vi "HFRR ADV v03.vi"() -> ()   [LabVIEW 2025] (continued)
            n287 = property on="Service Password Log" class="Str"("Visible"=FALSE) -> ()  [unwired: 2 in, 2 out]
            "Service Password enable" <- w384
          }
        }
      }
      event "Sign In": Value Change {
        w386 = FALSE ("Visible")
        n288 = event-data() -> ()  [unwired: 1 in, 6 out]
        n289 = property on="About" class="Clust (strict)"("Visible"=w386) -> ()  [unwired: 2 in, 2 out]
        n290 = property on="Password 3" class="Clust (strict)"("Visible"=w386) -> ()  [unwired: 2 in, 2 out]
        n291 = property on="Service Password Log" class="Str"("Visible"=FALSE) -> ()  [unwired: 2 in, 2 out]
      }
      event "Info": Value Change {
        n292 = event-data() -> ()  [unwired: 1 in, 6 out]
        n293 = local read "Info"() -> (w388:bool)
        n294 = case shown="False" w388 {
          frame False {
            n295 = property on="About" class="Clust (strict)"("Visible"=FALSE) -> ()  [unwired: 2 in, 2 out]
          }
          frame True {
            n296 = property on="About" class="Clust (strict)"("Visible"=TRUE) -> ()  [unwired: 2 in, 2 out]
          }
        }
      }
      event "Calibration": Value Change {
        n297 = event-data() -> ()  [unwired: 1 in, 6 out]
        n298 = local read "Calibration"() -> (w392:bool)
        n299 = case shown="False" w392 {
          frame False {
            n300 = property on="Calibration 2" class="TabCtl (strict)"("Visible"=FALSE) -> ()  [unwired: 2 in, 2 out]
            n301 = local write "Cal Password"("" ("Cal Password")) -> ()
          }
          frame True {
            n302 = property on="Calibration 2" class="TabCtl (strict)"("Visible"=TRUE) -> ()  [unwired: 2 in, 2 out]
            n303 = local write "Cal Password"("" ("Cal Password")) -> ()
          }
        }
        n304 = property on="Wrong Password" class="Str"("Visible"=FALSE) -> ()  [unwired: 2 in, 2 out]
      }
      event "Cal Password": Value Change {
        n305 = event-data() -> ()  [unwired: 1 in, 6 out]
        n306 = local read "Cal Password"() -> (w400:string)
        n307 = call <vilib>:"Trim Whitespace.vi"("string"=w400) -> ("trimmed string"=w399:string)  [unwired: 1 in]
        n308 = Equal?(x=w399, y="Cal@321") -> (x = y?=w397:bool)
        n309 = case shown="True" w397 {
          frame False {
            n310 = property on="Wrong Password" class="Str"("Visible"=TRUE) -> ()  [unwired: 2 in, 2 out]
          }
          frame True {
            n311 = property on="Wrong Password" class="Str"("Visible"=FALSE) -> ()  [unwired: 2 in, 2 out]
            n312 = local write "Main Tab"(T2."About" ("Main Tab")) -> ()
            n313 = local write "Cal Password"("" ("Cal Password")) -> ()
            n314 = local write "Main Dashboard Buttons"(T1."About" ("Main Dashboard Buttons")) -> ()
            n315 = local write "Tab Control 5"(T7."Temperature Calibration" ("Tab Control 5")) -> ()
            n316 = property on="Calibration 2" class="TabCtl (strict)"("Visible"=FALSE) -> ()  [unwired: 2 in, 2 out]
            n317 = property on="Tab Control 5" class="TabCtl (strict)"("Tabs Visible?"=FALSE ("Page Labels Display Visible?")) -> ()  [unwired: 2 in, 2 out]
            n318 = local write "Calibration"(FALSE ("Calibration")) -> ()
          }
        }
      }
      event "Quit": Value Change {
        n319 = event-data() -> ()  [unwired: 1 in, 6 out]
      }
    }
    n320 = Wait (ms)(milliseconds to wait=u32 100) -> ()  [unwired: 1 out]
  }
  n321 = local write "Auto stop temp"(w12) -> ()
  n322 = local write "main tab sub"(enum32{"Page 1", "Page 2"}."Page 1" ("main tab sub")) -> ()
  n323 = local write "USERNAME"(w31) -> ()
  n324 = local write "Main Tab"(T2."HOME" ("Main Tab")) -> ()
  n325 = local write "USER ID"(w31) -> ()
  n326 = property on="Auto Scar Check  2" class="Clust (strict)"("Visible"=w12) -> (error out=w16:errorcluster)  [unwired: 2 in, 1 out]
  n327 = property on="Quit" class="Bool (strict)"("Value"=FALSE ("Quit")) -> (error out=w33:errorcluster)  [unwired: 2 in, 1 out]
  n328 = while {
    shift-right: [w412] -> _
    shift-left: "Enum - Selector" -> [w413]
    stop <- w414 stop-if-true
    # "Auto Start Logic Loop"
    n329 = case shown="\"close\"" w413 {
      tunnel: [w417 w423 w434 w466 w497 Auto_Start_enum."Exit" ("Enum - Selector") Auto_Start_enum."Init" ("Enum - Selector")] -> w412
      frame "Init", Default {
        n330 = local read "Auto Start Test"() -> (w416:bool)
        n331 = Select(t=Auto_Start_enum."Humidity & Temperature On" ("Enum - Selector"), s=w416, f=Auto_Start_enum."Init") -> (s? t:f=w417:T10)
      }
      frame "Humidity & Temperature On" {
        n332 = flat-sequence {
          tunnel: [Auto_Start_enum."Reach point" ("Enum - Selector")] -> w420
          frame #0 {
            w424 = T13."Disabled and Grayed Out" ("Disabled")
            w425 = TRUE ("Heater Button")
            n333 = property on="Humidity" class="Bool (strict)"("DisabledEnum"=w424) -> ()  [unwired: 2 in, 2 out]
            n334 = property on="Heater Button" class="Bool (strict)"("DisabledEnum"=w424) -> ()  [unwired: 2 in, 2 out]
            n335 = local write "Heater Button"(w425) -> ()
            n336 = local write "Humidity"(w425) -> ()
          }
          frame #1 {
            n337 = Wait (ms)(milliseconds to wait=u32 1000) -> ()  [unwired: 1 out]
          }
          frame #2 {
            w427 = TRUE ("Reach point temp")
            n338 = local write "Reach point Humidity"(w427) -> ()
            n339 = local write "Reach point temp"(w427) -> ()
          }
        }
        n340 = local read "Auto Start Test"() -> (w422:bool)
        n341 = Not(x=w422) -> (.not. x?=w421:bool)
        n342 = Select(t=Auto_Start_enum."close", s=w421, f=w420) -> (s? t:f=w423:T10)
      }
      frame "Reach point" {
        w435 = TRUE ("PAUSE")
        w443 = 1.0 ("y")
        w446 = 1.0 ("y")
        n343 = local read "Set Temperature:"() -> (w447:dbl)
        n344 = local read "Set Humidity:"() -> (w442:dbl)
        n345 = local read "Humidity ( %RH )"() -> (w448:dbl)
        n346 = Add(x=w447, y=w446) -> (x+y=w445:dbl)
        n347 = Subtract(x=w447, y=w446) -> (x-y=w444:dbl)
        n348 = Add(x=w442, y=w443) -> (x+y=w441:dbl)
        n349 = Subtract(x=w442, y=w443) -> (x-y=w440:dbl)
        n350 = local read "TEMP"() -> (w449:dbl)
        n351 = In Range and Coerce(upper limit=w441, x=w448, lower limit=w440) -> (In Range?=w429:bool)  [unwired: 1 out]
        n352 = In Range and Coerce(upper limit=w445, x=w449, lower limit=w444) -> (In Range?=w430:bool)  [unwired: 1 out]
        n353 = case shown="True" w429 {
          frame False {
          }
          frame True {
            n354 = case shown="True" "Reach point Humidity" {
              selector: "Reach point Humidity" -> [_ w455]
              frame False {
              }
              frame True {
                n355 = local read "EVENT LOG"() -> (w452:string)
                n356 = Not(x=w455) -> (.not. x?=w454:bool)
                n357 = local write "Reach point Humidity"(w454) -> ()
                n358 = call "Event Log.vi"("Content"="Target Humidity reached", "EVENT LOG"=w452) -> ("EVENT LOG"=w453:string)  [unwired: 8 in, 1 out]
                n359 = local write "EVENT LOG"(w453) -> ()
              }
            }
          }
        }
        n360 = case shown="True" w430 {
          frame False {
          }
          frame True {
            n361 = case shown="True" "Reach point temp" {
              selector: "Reach point temp" -> [_ w461]
              frame False {
              }
              frame True {
                n362 = local read "EVENT LOG"() -> (w458:string)
                n363 = Not(x=w461) -> (.not. x?=w460:bool)
                n364 = local write "Reach point temp"(w460) -> ()
                n365 = call "Event Log.vi"("Content"="Target Temperature reached", "EVENT LOG"=w458) -> ("EVENT LOG"=w459:string)  [unwired: 8 in, 1 out]
                n366 = local write "EVENT LOG"(w459) -> ()
              }
            }
          }
        }
        n367 = local read "Auto Start Test"() -> (w433:bool)
        n368 = And(x=w430, y=w429) -> (x .and. y?=w439:bool)
        n369 = Select(t=Auto_Start_enum."Maintain Stage" ("Enum - Selector"), s=w439, f=Auto_Start_enum."Reach point" ("Enum - Selector")) -> (s? t:f=w436:T10)
        n370 = Not(x=w433) -> (.not. x?=w432:bool)
        n371 = Select(t=Auto_Start_enum."close", s=w432, f=w436) -> (s? t:f=w434:T10)
        n372 = call "ELAPSED TIMER VI.vi"("RESET"=w435, "PAUSE"=w435) -> ()  [unwired: 7 in, 3 out]
      }
      frame "Maintain Stage" {
        w475 = 2.0 ("y")
        w474 = 1.0 ("y")
        # "Humidity and  temperatures Set Point  have been reached"
        n373 = local read "Set Temperature:"() -> (w481:dbl)
        n374 = local read "Set Humidity:"() -> (w478:dbl)
        n375 = local read "Humidity ( %RH )"() -> (w482:dbl)
        n376 = Add(x=w481, y=w474) -> (x+y=w480:dbl)
        n377 = Subtract(x=w481, y=w474) -> (x-y=w479:dbl)
        n378 = local read "TEMP"() -> (w483:dbl)
        n379 = Add(x=w478, y=w475) -> (x+y=w477:dbl)
        n380 = Subtract(x=w478, y=w475) -> (x-y=w476:dbl)
        n381 = In Range and Coerce(upper limit=w480, x=w483, lower limit=w479) -> (In Range?=w473:bool)  [unwired: 1 out]
        n382 = In Range and Coerce(upper limit=w477, x=w482, lower limit=w476) -> (In Range?=w472:bool)  [unwired: 1 out]
        n383 = And(x=w473, y=w472) -> (x .and. y?=w471:bool)
        n384 = Not(x=w471) -> (.not. x?=w470:bool)
        n385 = call "ELAPSED TIMER VI.vi"("TARGET"=60.0, "RESET"=w470, "PAUSE"=FALSE) -> ("ELAPSED INDICATION"=w467:bool)  [unwired: 6 in, 2 out]
        n386 = case shown="True" w467 {
          tunnel: w467 -> [_ w486]
          tunnel: [Auto_Start_enum."Maintain Stage" ("Enum - Selector") w485] -> w465
          frame False {
          }
          frame True {
            n387 = stacked-sequence {
              tunnel: w486 -> [_ _ _ _ _]
              tunnel: [_ _ _ _ Auto_Start_enum."Start Stage" ("Enum - Selector")] -> w485
              frame #0 {
                n388 = local read "EVENT LOG"() -> (w488:string)
                n389 = call "Event Log.vi"("Content"="Humidity and temperature set point has stabilized.", "EVENT LOG"=w488) -> ("EVENT LOG"=w489:string)  [unwired: 8 in, 1 out]
                n390 = local write "EVENT LOG"(w489) -> ()
              }
              frame #1 {
                n391 = Wait (ms)(milliseconds to wait=u32 100) -> ()  [unwired: 1 out]
              }
              frame #2 {
                n392 = local read "EVENT LOG"() -> (w492:string)
                n393 = call "Event Log.vi"("Content"="Auto Test Started", "EVENT LOG"=w492) -> ("EVENT LOG"=w493:string)  [unwired: 8 in, 1 out]
                n394 = local write "EVENT LOG"(w493) -> ()
              }
              frame #3 {
                w494 = TRUE ("RUN")
                n395 = local write "RUN"(w494) -> ()
                "Auto Start Temp" <- w494
              }
              frame #4 {
              }
            }
          }
        }
        n396 = local read "Auto Start Test"() -> (w464:bool)
        n397 = Not(x=w464) -> (.not. x?=w463:bool)
        n398 = Select(t=Auto_Start_enum."close", s=w463, f=w465) -> (s? t:f=w466:T10)
      }
      frame "Start Stage" {
        w496 = TRUE ("PAUSE")
        n399 = local read "Auto Start Test"() -> (w501:bool)
        n400 = Not(x=w501) -> (.not. x?=w500:bool)
        n401 = Select(t=Auto_Start_enum."close" ("Enum - Selector"), s=w500, f=Auto_Start_enum."Start Stage" ("Enum - Selector")) -> (s? t:f=w497:T10)
        n402 = call "ELAPSED TIMER VI.vi"("RESET"=w496, "PAUSE"=w496) -> ()  [unwired: 7 in, 3 out]
      }
      frame "close" {
        w502 = FALSE ("Heater Button")
        n403 = local write "RUN"(w502) -> ()
        n404 = local write "Heater Button"(w502) -> ()
        n405 = local write "Humidity"(w502) -> ()
        n406 = local write "Auto Start Test"(w502) -> ()
      }
      frame "Exit" {
      }
    }
    n407 = Wait (ms)(milliseconds to wait=u32 100) -> ()  [unwired: 1 out]
    n408 = local read "Quit"() -> (w414:bool)
  }
  n409 = while {
    stop <- w531 stop-if-true
    w514 = errorcluster {"status"=FALSE, "code"=0, "source"=""} ("error in (no error) 3")
    # "this loop is for manual report generation"
    n410 = local read "Confirm Measrurement"() -> (w513:bool)
    n411 = case shown="True" w513 {
      selector: w513 -> [_ w621]
      tunnel: errorcluster {"status"=FALSE, "code"=0, "source"=""} ("error in (no error) 3") -> [_ w622]
      tunnel: [_ w620] -> _
      frame False {
      }
      frame True {
        n412 = stacked-sequence {
          tunnel: w622 -> [_ w655 _]
          tunnel: w621 -> [_ _ w762]
          tunnel: [_ w643 _] -> w620
          frame #0 {
            n413 = String To Path(string="C:\\LAB-IQ\\Image Calibrate v01.dcf") -> (path=w625:path)
            n414 = Open/Create/Replace File ("Open File")(file path (use dialog)=w625) -> (refnum out=w626:refnum<file>)  [unwired: 5 in, 2 out]
            n415 = for {
              N: 4 -> [_]
              tunnel: w626 -> [w632]
              i -> [w628]
              n416 = Read from Text File ("Read File")(file (use dialog)=w632) -> (text=w633:string)  [unwired: 3 in, 3 out]
              n417 = String Subset(string=w633, offset (0)=6, length (rest)=10 ("length (rest)")) -> (substring=w629:string)
              n418 = Fract/Exp String To Number(string=w629) -> (number=w627:dbl)  [unwired: 3 in, 1 out]
              n419 = case shown="3" w628 {
                tunnel: w627 -> [w634 w635 _ w636 _]
                frame 0 {
                  n420 = local write "5x Gain"(w634) -> ()
                }
                frame 1 {
                  n421 = local write "10x Gain"(w635) -> ()
                }
                frame 2 {
                }
                frame 3 {
                  n422 = local write "100x gain"(w636) -> ()
                }
                frame 4, Default {
                }
              }
            }
          }
          frame #1 {
            n423 = local read "TEST STANDARD"() -> (w638:T3)
            n424 = case shown="\"ISO 12156\"" w638 {
              tunnel: ["ASTM D6079" "ISO 12156"] -> w637
              frame "ASTM D6079", Default {
              }
              frame "ISO 12156" {
              }
            }
            n425 = call "IMAGE ANALYSIS.vi"("Enum"=POST_ANALYSIS_ENUM."GET MEASUREMENTS", "error in"=w655) -> ("error out"=w662:errorcluster)  [unwired: 8 in, 1 out]
            n426 = local read "Magnification :"() -> (w648:string)
            n427 = call "Stall Data Flow.vim"("value in"=w662, "milliseconds to wait"=u32 1000) -> ("value out"=w661:errorcluster)  [unwired: 1 out]
            n428 = local read "Test File List :"() -> (w659:string)
            n429 = case shown="\"10x\"" w648 {
              tunnel: [w698 w699] -> w646
              frame "5x", Default {
                n430 = local read "5x Gain"() -> (w698:dbl)
              }
              frame "10x" {
                # "5x"
                n431 = local read "10x Gain"() -> (w699:dbl)
              }
            }
            n432 = call "IMAGE ANALYSIS.vi"("Enum"=POST_ANALYSIS_ENUM."READ", "error in"=w661) -> ("error out"=w658:errorcluster, "data out"=w649:string)  [unwired: 8 in]
            n433 = Match Pattern(string=w649, regular expression="\"type\": ") -> (after substring=w653:string)  [unwired: 1 in, 3 out]
            n434 = call "IMAGE PATH CREATION PY.vi"("error in (no error)"=w658, "File Name :"=w659) -> ("error out"=w657:errorcluster, "File Path"=w645:path, "File Path String:"=w640:string)  [unwired: 7 in]
            n435 = Match Pattern(string=w653, regular expression=",") -> (before substring=w639:string)  [unwired: 1 in, 3 out]
            n436 = local read "Calibration Tab"() -> (w642:enum32{"Measrument", "Calibrate"})
            n437 = call "Stall Data Flow.vim"("value in"=w657, "milliseconds to wait"=u32 250) -> ("value out"=w641:errorcluster)  [unwired: 1 out]
            n438 = Equal?(x=w639, y="\"rectangle\"") -> (x = y?=w650:bool)
            n439 = case shown="False" w650 {
              tunnel: w649 -> [w704 w759]
              tunnel: w646 -> [_ w750]
              tunnel: cluster{"major":dbl, "minor":dbl, "average":dbl} {"major"=0.0, "minor"=0.0, "average"=0.0} -> [w702 w746]
              tunnel: [w701 w743] -> w644
              tunnel: w639 -> [w703 _]
              tunnel: w646 -> [w700 _]
              frame False {
                n440 = Equal?(x=w703, y="\"line\"") -> (x = y?=w705:bool)
                n441 = case shown="True" w705 {
                  tunnel: w704 -> [_ w720]
                  tunnel: w702 -> [w707 w719]
                  tunnel: [w707 w717] -> w701
                  tunnel: w700 -> [_ w716]
                  frame False {
                  }
                  frame True {
                    w715 = 0.0 ("Major Axis")
                    n442 = Match Pattern(string=w720, regular expression="\"length_px\":") -> (after substring=w718:string)  [unwired: 1 in, 3 out]
                    n443 = property on="Major Axis" class="DigNum (strict)"("Caption.Text"="") -> ()  [unwired: 2 in, 2 out]
                    n444 = property on="Minor Axis" class="DigNum (strict)"("Caption.Text"="") -> ()  [unwired: 2 in, 2 out]
                    n445 = property on="Average" class="DigNum (strict)"("Caption.Text"="Line") -> ()  [unwired: 2 in, 2 out]
                    n446 = Fract/Exp String To Number(string=w718, default (0 dbl)=0.0 ("default (0 DBL)")) -> (number=w714:dbl)  [unwired: 2 in, 1 out]
                    "Pixel Value" <- w714
                    n447 = Multiply(x=w714, y=w716) -> (x*y=w727:dbl)
                    n448 = Multiply(x=w727, y=1000.0) -> (x*y=w710:dbl)
                    n449 = Divide(x=w710, y=1000.0) -> (x/y=w713:dbl)
                    n450 = local write "Measurment (mm)"(w713) -> ()
                    n451 = Bundle By Name(cluster=w719, "average"=w710) -> (w717:cluster{"major":dbl, "minor":dbl, "average":dbl})
                    n452 = Number To Fractional String(number=w710, precision (6)=i16 1) -> (F-format string=w709:string)  [unwired: 2 in]
                    n453 = local write "Minor Axis"(w715) -> ()
                    n454 = local write "Major Axis"(w715) -> ()
                    n455 = Fract/Exp String To Number(string=w709) -> (number=w708:dbl)  [unwired: 3 in, 1 out]
                    n456 = local write "Average"(w708) -> ()
                  }
                }
              }
              frame True {
                w747 = 1000.0 ("y")
                w753 = 0.0 ("default (0 DBL)")
                n457 = Match Pattern(string=w759, regular expression=" \"width_px\":") -> (after substring=w757:string)  [unwired: 1 in, 3 out]
                n458 = Match Pattern(string=w757, regular expression="\"height_px\":") -> (before substring=w755:string, after substring=w754:string)  [unwired: 1 in, 2 out]
                n459 = Fract/Exp String To Number(string=w755, default (0 dbl)=w753) -> (number=w752:dbl)  [unwired: 2 in, 1 out]
                n460 = Fract/Exp String To Number(string=w754, default (0 dbl)=w753) -> (number=w751:dbl)  [unwired: 2 in, 1 out]
                n461 = Multiply(x=w752, y=w750) -> (x*y=w749:dbl)
                n462 = Multiply(x=w751, y=w750) -> (x*y=w748:dbl)
                n463 = Multiply(x=w749, y=w747) -> (x*y=w733:dbl)
                n464 = Multiply(x=w748, y=w747) -> (x*y=w731:dbl)
                n465 = Add(x=w733, y=w731) -> (x+y=w745:dbl)
                n466 = property on="Major Axis" class="DigNum (strict)"("Caption.Text"="Major Axis") -> ()  [unwired: 2 in, 2 out]
                n467 = property on="Minor Axis" class="DigNum (strict)"("Caption.Text"="Minor Axis") -> ()  [unwired: 2 in, 2 out]
                n468 = property on="Average" class="DigNum (strict)"("Caption.Text"="Average") -> ()  [unwired: 2 in, 2 out]
                n469 = Divide(x=w745, y=2.0) -> (x/y=w729:dbl)
                n470 = Bundle By Name(cluster=w746, "major"=w733, "minor"=w731, "average"=w729) -> (w743:cluster{"major":dbl, "minor":dbl, "average":dbl})
                n471 = Number To Fractional String(number=w731, precision (6)=i16 1) -> (F-format string=w738:string)  [unwired: 2 in]
                n472 = Number To Fractional String(number=w729, precision (6)=i16 1) -> (F-format string=w739:string)  [unwired: 2 in]
                n473 = Number To Fractional String(number=w733, precision (6)=i16 1) -> (F-format string=w737:string)  [unwired: 2 in]
                n474 = Fract/Exp String To Number(string=w738) -> (number=w730:dbl)  [unwired: 3 in, 1 out]
                n475 = Fract/Exp String To Number(string=w739) -> (number=w728:dbl)  [unwired: 3 in, 1 out]
                n476 = Fract/Exp String To Number(string=w737) -> (number=w732:dbl)  [unwired: 3 in, 1 out]
                n477 = local write "Major Axis"(w732) -> ()
                n478 = local write "Average"(w728) -> ()
                n479 = local write "Minor Axis"(w730) -> ()
              }
            }
            n480 = case shown="\"Measrument\", Default" w642 {
              tunnel: w645 -> [w672 _]
              tunnel: w644 -> [w671 _]
              tunnel: [w668 w697] -> w643
              tunnel: w641 -> [w670 w697]
              tunnel: w640 -> [w669 _]
              tunnel: w637 -> [w667 _]
              frame "Measrument", Default {
                n481 = stacked-sequence {
                  tunnel: w672 -> [w690 _]
                  tunnel: w671 -> [w688 _]
                  tunnel: w670 -> [w686 _]
                  tunnel: w669 -> [w685 _]
                  tunnel: [w680 _] -> w668
                  tunnel: w667 -> [w673 _]
                  frame #0 {
                    n482 = call "IMAGE ANALYSIS.vi"("Enum"=POST_ANALYSIS_ENUM."SAVE IMAGE", "error in"=w686, "IMAGE FILE PATH"=w685) -> ("error out"=w684:errorcluster)  [unwired: 7 in, 1 out]
                    n483 = call "Stall Data Flow.vim"("value in"=w684, "milliseconds to wait"=u32 1000) -> ("value out"=w675:errorcluster)  [unwired: 1 out]
                    n484 = local read "Test File List :"() -> (w692:string)
                    n485 = call "IMAGE ANALYSIS.vi"("Enum"=POST_ANALYSIS_ENUM."MINIMIZE UI", "error in"=w675) -> ("error out"=w682:errorcluster)  [unwired: 8 in, 1 out]
                    n486 = Bundle By Name(cluster=T18 {"File Name"="", "Test Method"="", "Operator"="", "Fuel Description"="", "Date and time"=""} ("Main Ref"), "Test Method"=w673, "File Name"=w692) -> (w693:T18)
                    n487 = call "Stall Data Flow.vim"("value in"=w682, "milliseconds to wait"=u32 1500) -> ("value out"=w677:errorcluster)  [unwired: 1 out]
                    n488 = call "duf file read.vi"("error in (no error)"=w677, "Main Ref"=w693) -> ("error out"=w691:errorcluster, "Main Ref 2"=w689:T18)  [unwired: 8 in]
                    n489 = call "DETECTION REPORT for manual.vi"("error in (no error)"=w691, "return value 3"=w688, "Image File Path"=w690, "Main Ref"=w689) -> ("error out"=w687:errorcluster)  [unwired: 7 in]
                    n490 = call <vilib>:"Clear Errors.vi"("error in (no error)"=w687) -> ("error out"=w678:errorcluster)  [unwired: 5 in, 1 out]
                    n491 = call "IMAGE ANALYSIS.vi"("Enum"=POST_ANALYSIS_ENUM."MINIMIZE UI", "error in"=w678) -> ("error out"=w680:errorcluster)  [unwired: 8 in, 1 out]
                  }
                  frame #1 {
                    n492 = local write "Main Tab"(T2."HOME" ("Main Tab")) -> ()
                    n493 = local write "Main Dashboard Buttons"(T1."Home" ("Main Dashboard Buttons")) -> ()
                  }
                }
              }
              frame "Calibrate" {
              }
            }
          }
          frame #2 {
            n494 = Not(x=w762) -> (.not. x?=w761:bool)
            n495 = local write "Confirm Measrurement"(w761) -> ()
            n496 = local read "Calibration Tab"() -> (w760:enum32{"Measrument", "Calibrate"})
            n497 = case shown="\"Measrument\", Default" w760 {
              frame "Measrument", Default {
                n498 = local write "Main Tab"(T2."HOME" ("Main Tab")) -> ()
              }
              frame "Calibrate" {
              }
            }
          }
        }
      }
    }
    n499 = local read "Humidity"() -> (w505:bool)
    n500 = local read "Save Change"() -> (w510:bool)
    n501 = local read "Calibrate"() -> (w511:bool)
    n502 = local read "Auto Start Test"() -> (w506:bool)
    n503 = case shown="True" w511 {
      selector: w511 -> [_ w618]
      frame False {
      }
      frame True {
        n504 = Not(x=w618) -> (.not. x?=w617:bool)
        n505 = local write "Calibrate"(w617) -> ()
        n506 = local write "Calibration Tab"(enum32{"Measrument", "Calibrate"}."Calibrate" ("Calibration Tab")) -> ()
      }
    }
    n507 = case shown="True" w510 {
      selector: w510 -> [_ w562]
      frame False {
      }
      frame True {
        n508 = stacked-sequence {
          tunnel: w562 -> [_ _ _ _ w616]
          frame #0 {
            n509 = call "IMAGE ANALYSIS.vi"("Enum"=POST_ANALYSIS_ENUM."HIDE UI") -> ()  [unwired: 9 in, 2 out]
          }
          frame #1 {
            n510 = local read "100x gain"() -> (w564:dbl)
            n511 = local read "10x Gain"() -> (w565:dbl)
            n512 = local read "5x Gain"() -> (w566:dbl)
            n513 = Number To Fractional String(number=w565, width (-)=i16 4, precision (6)=i16 7) -> (F-format string=w587:string)  [unwired: 1 in]
            n514 = Number To Fractional String(number=0.0, width (-)=i16 4, precision (6)=i16 7) -> (F-format string=w582:string)  [unwired: 1 in]
            n515 = Number To Fractional String(number=w564, width (-)=i16 4, precision (6)=i16 7) -> (F-format string=w570:string)  [unwired: 1 in]
            n516 = Number To Fractional String(number=w566, width (-)=i16 10 ("precision (6)"), precision (6)=i16 7) -> (F-format string=w596:string)  [unwired: 1 in]
            n517 = Concatenate Strings("[CH1]" ("string"), w596, " - 5x Gain" ("string"), "\r") -> (w586:string)
            n518 = Concatenate Strings("[CH2]" ("string"), w587, " - 10x Gain" ("string"), "\r") -> (w585:string)
            n519 = Concatenate Strings("[CH3]" ("string"), w582, " - 20x Gain" ("string"), "\r") -> (w576:string)
            n520 = Concatenate Strings("[CH4]" ("string"), w570, " - 100x Gain" ("string"), "\r") -> (w569:string)
            n521 = String To Path(string="C:\\LAB-IQ\\Image Calibrate v01.dcf") -> (path=w599:path)
            n522 = Concatenate Strings(w586, w585, w576, w569) -> (w584:string)
            n523 = call <vilib>:"Write Characters To File.vi"("append to file? (new file:F)"=FALSE, "character string"=w584, "file path (dialog if empty)"=w599) -> ()  [unwired: 2 in, 1 out]
          }
          frame #2 {
            n524 = String To Path(string="C:\\LAB-IQ\\Image Calibrate v01.dcf") -> (path=w602:path)
            n525 = Open/Create/Replace File ("Open File")(file path (use dialog)=w602) -> (refnum out=w603:refnum<file>)  [unwired: 5 in, 2 out]
            n526 = for {
              N: 4 -> [_]
              tunnel: w603 -> [w609]
              i -> [w605]
              n527 = Read from Text File ("Read File")(file (use dialog)=w609) -> (text=w610:string)  [unwired: 3 in, 3 out]
              n528 = String Subset(string=w610, offset (0)=6, length (rest)=10 ("length (rest)")) -> (substring=w606:string)
              n529 = Fract/Exp String To Number(string=w606) -> (number=w604:dbl)  [unwired: 3 in, 1 out]
              n530 = case shown="3" w605 {
                tunnel: w604 -> [w611 w612 _ w613 _]
                frame 0 {
                  n531 = local write "5x Gain"(w611) -> ()
                }
                frame 1 {
                  n532 = local write "10x Gain"(w612) -> ()
                }
                frame 2 {
                }
                frame 3 {
                  n533 = local write "100x gain"(w613) -> ()
                }
                frame 4, Default {
                }
              }
            }
          }
          frame #3 {
            n534 = call "IMAGE ANALYSIS.vi"("Enum"=POST_ANALYSIS_ENUM."SHOW UI") -> ()  [unwired: 9 in, 2 out]
          }
          frame #4 {
            n535 = Not(x=w616) -> (.not. x?=w615:bool)
            n536 = local write "Save Change"(w615) -> ()
          }
        }
      }
    }
    n537 = case shown="False" w506 {
      tunnel: w505 -> [w532 _]
      frame False {
        n538 = case shown="True" w532 {
          frame False {
          }
          frame True {
            n539 = local read "Set Humidity:"() -> (w536:dbl)
            n540 = local read "Set Humidity:"() -> (w539:dbl)
            n541 = local read "Humidity ( %RH )"() -> (w540:dbl)
            n542 = Subtract(x=w536, y=2.0) -> (x-y=w534:dbl)
            n543 = Add(x=w539, y=2.0) -> (x+y=w535:dbl)
            n544 = In Range and Coerce(upper limit=w535, x=w540, lower limit=w534) -> (In Range?=w533:bool)  [unwired: 1 out]
            n545 = case shown="True" w533 {
              frame False {
              }
              frame True {
                n546 = case shown="False" "Manual Humididty Reached" {
                  selector: "Manual Humididty Reached" -> [_ w543]
                  frame False {
                  }
                  frame True {
                    n547 = Not(x=w543) -> (.not. x?=w542:bool)
                    n548 = local write "Manual Humididty Reached"(w542) -> ()
                    n549 = local read "EVENT LOG"() -> (w545:string)
                    n550 = call "Event Log.vi"("Content"="Target Humidity reached", "EVENT LOG"=w545) -> ("EVENT LOG"=w544:string)  [unwired: 8 in, 1 out]
                    n551 = local write "EVENT LOG"(w544) -> ()
                  }
                }
              }
            }
          }
        }
      }
      frame True {
        n552 = local write "Manual Humididty Reached"(TRUE ("Manual Humididty Reached")) -> ()
      }
    }
    n553 = local read "Cap Live Image"() -> (w526:bool)
    n554 = local read "SCAR MEASURMENT"() -> (w529:enum32{"Auto Scar", "Manual Scar"})
    n555 = Wait (ms)(milliseconds to wait=u32 250) -> ()  [unwired: 1 out]
    n556 = Equal?(x=w529, y=enum32{"Auto Scar", "Manual Scar"}."Manual Scar" ("SCAR MEASURMENT")) -> (x = y?=w527:bool)
    n557 = And(x=w527, y=w526) -> (x .and. y?=w525:bool)
    n558 = case shown="True" w525 {
      selector: w525 -> [_ w841]
      frame False {
      }
      frame True {
        n559 = stacked-sequence {
          tunnel: [_ _ _ w856 _] -> _
          tunnel: w841 -> [_ _ _ _ w862]
          frame #0 {
            w842 = 0.0
            n560 = local write "Major Axis"(w842) -> ()
            n561 = local write "Minor Axis"(w842) -> ()
            n562 = local write "Average"(w842) -> ()
          }
          frame #1 {
            n563 = call "CAMERA LIVE FEED FGV.vi"("Enum - Menu"=CAMERA_LIVE_FEED_ENUM."CAMERA MINIMIZE") -> ()  [unwired: 9 in, 2 out]
          }
          frame #2 {
            n564 = local read "FILE 3"() -> (w850:string)
            n565 = call <vilib>:"Trim Whitespace.vi"("string"="C:\\LAB-IQ\\images\\") -> ("trimmed string"=w852:string)  [unwired: 1 in]
            n566 = String To Path(string=w852) -> (path=w851:path)
            n567 = Concatenate Strings(w850, ".png" ("string")) -> (w849:string)
            n568 = Build Path(base path=w851, name or relative path=w849) -> (appended path=w847:path)
            n569 = Path To String(path=w847) -> (string=w846:string)
            n570 = call "CAMERA LIVE FEED FGV.vi"("Enum - Menu"=CAMERA_LIVE_FEED_ENUM."CAMERA SAVE", "Image Path"=w846) -> ("error out"=w844:errorcluster)  [unwired: 8 in, 1 out]
            n571 = case shown="No Error" w844 {
              frame No Error {
                n572 = One Button Dialog(message="Image saved successfully") -> ()  [unwired: 1 in, 1 out]
              }
              frame Error {
              }
            }
          }
          frame #3 {
            n573 = call "LIST FILE NAMES.vi"() -> ("error out"=w858:errorcluster, "filenames"=w855:string[])  [unwired: 10 in]
            n574 = call "IMAGE ANALYSIS.vi"("Enum"=POST_ANALYSIS_ENUM."SHOW UI", "error in"=w858) -> ("error out"=w856:errorcluster)  [unwired: 8 in, 1 out]
            n575 = property on="Test File List :" class="CmbBox"("Strings[]"=w855) -> ()  [unwired: 2 in, 2 out]
          }
          frame #4 {
            (unwired) T19."Report" ("Main Dashboard Buttons")
            n576 = Not(x=w862) -> (.not. x?=w861:bool)
            n577 = local write "Zoom Factore"(0.0 ("Zoom Factore")) -> ()
            n578 = local write "Cap Live Image"(w861) -> ()
            n579 = local write "Main Tab"(T2."Adv Scar Report" ("Main Tab")) -> ()
            n580 = property on="Cap Live Image" class="Bool (strict)"("BoolText.Text"="Capture Image" ("Boolean Text.Text")) -> ()  [unwired: 2 in, 2 out]
            n581 = local write "Main Dashboard Buttons"(T1."Report" ("Main Dashboard Buttons")) -> ()
          }
        }
      }
    }
    n582 = local read "change Gain"() -> (w509:bool)
    n583 = local read "Back Square"() -> (w508:bool)
    n584 = case shown="True" w509 {
      selector: w509 -> [_ w553]
      frame False {
      }
      frame True {
        n585 = stacked-sequence {
          tunnel: w553 -> [_ w561]
          frame #0 {
            n586 = local read "Actual (µm)"() -> (w557:dbl)
            n587 = local read "Pixel Value"() -> (w556:dbl)
            n588 = local read "Magnification :"() -> (w555:string)
            n589 = Divide(x=w557, y=w556) -> (x/y=w554:dbl)
            n590 = case shown="\"10x\"" w555 {
              tunnel: w554 -> [w558 w559]
              frame "10x" {
                n591 = local write "10x Gain"(w558) -> ()
              }
              frame "5x", Default {
                n592 = local write "5x Gain"(w559) -> ()
              }
            }
          }
          frame #1 {
            n593 = Not(x=w561) -> (.not. x?=w560:bool)
            n594 = local write "change Gain"(w560) -> ()
          }
        }
      }
    }
    n595 = case shown="True" w508 {
      selector: w508 -> [_ w551]
      frame False {
      }
      frame True {
        n596 = Not(x=w551) -> (.not. x?=w550:bool)
        n597 = local write "Back Square"(w550) -> ()
        n598 = local write "Calibration Tab"(enum32{"Measrument", "Calibrate"}."Measrument" ("Calibration Tab")) -> ()
      }
    }
    n599 = local read "Rectangle Tool"() -> (w520:bool)
    n600 = local read "Clear ROI Tool"() -> (w519:bool)
    n601 = local read "Open Image"() -> (w524:bool)
    n602 = local read "line tool"() -> (w521:bool)
    n603 = local read "OUT"() -> (w522:bool)
    n604 = local read "In"() -> (w523:bool)
    n605 = case shown="True" w524 {
      selector: w524 -> [_ w829]
      tunnel: [w825 w831] -> _
      tunnel: w514 -> [w825 w830]
      frame False {
      }
      frame True {
        n606 = Not(x=w829) -> (.not. x?=w828:bool)
        n607 = local write "Open Image"(w828) -> ()
        n608 = call "IMAGE ANALYSIS.vi"("Enum"=POST_ANALYSIS_ENUM."HIDE UI", "error in"=w830) -> ("error out"=w838:errorcluster)  [unwired: 8 in, 1 out]
        n609 = call "File Dialog"("start path"=path "C:/LAB-IQ/images", "error in"=w838) -> ("selected path"=w827:path, "error out"=w836:errorcluster)  [unwired: 10 in, 2 out]
        "Image path  2" <- w827
        n610 = call <vilib>:"Clear Errors.vi"("error in (no error)"=w836) -> ("error out"=w835:errorcluster)  [unwired: 5 in, 1 out]
        n611 = call "IMAGE ANALYSIS.vi"("Enum"=POST_ANALYSIS_ENUM."OPEN FILE", "error in"=w835, "File Path"=w827) -> ("error out"=w834:errorcluster)  [unwired: 7 in, 1 out]
        n612 = call <vilib>:"Clear Errors.vi"("error in (no error)"=w834) -> ("error out"=w833:errorcluster)  [unwired: 5 in, 1 out]
        n613 = call "IMAGE ANALYSIS.vi"("Enum"=POST_ANALYSIS_ENUM."SHOW UI", "error in"=w833) -> ("error out"=w831:errorcluster)  [unwired: 8 in, 1 out]
        n614 = local write "Zoom Factore"(100.0 ("Zoom Factore")) -> ()
      }
    }
    n615 = case shown="True" w522 {
      selector: w522 -> [_ w810]
      tunnel: w514 -> [w807 w815]
      tunnel: [w807 w809] -> _
      frame False {
      }
      frame True {
        n616 = Not(x=w810) -> (.not. x?=w808:bool)
        n617 = local read "Zoom Factore"() -> (w813:dbl)
        n618 = local write "OUT"(w808) -> ()
        n619 = call "IMAGE ANALYSIS.vi"("Enum"=POST_ANALYSIS_ENUM."ZOOM OUT", "error in"=w815) -> ("error out"=w809:errorcluster)  [unwired: 8 in, 1 out]
        n620 = Divide(x=w813, y=1.2) -> (x/y=w811:dbl)
        n621 = local write "Zoom Factore"(w811) -> ()
      }
    }
    n622 = case shown="True" w523 {
      selector: w523 -> [_ w819]
      tunnel: w514 -> [w816 w824]
      tunnel: [w816 w817] -> _
      frame False {
      }
      frame True {
        n623 = Not(x=w819) -> (.not. x?=w818:bool)
        n624 = local read "Zoom Factore"() -> (w822:dbl)
        n625 = local write "In"(w818) -> ()
        n626 = call "IMAGE ANALYSIS.vi"("Enum"=POST_ANALYSIS_ENUM."ZOOM IN", "error in"=w824) -> ("error out"=w817:errorcluster)  [unwired: 8 in, 1 out]
        n627 = Multiply(x=w822, y=1.2) -> (x*y=w820:dbl)
        n628 = local write "Zoom Factore"(w820) -> ()
      }
    }
    n629 = case shown="True" w519 {
      selector: w519 -> [_ w791]
      tunnel: w514 -> [w789 w793]
      tunnel: [w789 w792] -> _
      frame False {
      }
      frame True {
        n630 = Not(x=w791) -> (.not. x?=w790:bool)
        n631 = local write "Clear ROI Tool"(w790) -> ()
        n632 = call "IMAGE ANALYSIS.vi"("Enum"=POST_ANALYSIS_ENUM."CLEAR ROI", "error in"=w793) -> ("error out"=w792:errorcluster)  [unwired: 8 in, 1 out]
      }
    }
    n633 = case shown="True" w521 {
      selector: w521 -> [_ w803]
      tunnel: w514 -> [w801 w806]
      tunnel: [w801 w804] -> _
      frame False {
      }
      frame True {
        n634 = Not(x=w803) -> (.not. x?=w802:bool)
        n635 = local write "line tool"(w802) -> ()
        n636 = call "IMAGE ANALYSIS.vi"("Enum"=POST_ANALYSIS_ENUM."DRAW LINE", "error in"=w806) -> ("error out"=w804:errorcluster)  [unwired: 8 in, 1 out]
      }
    }
    n637 = case shown="True" w520 {
      selector: w520 -> [_ w797]
      tunnel: w514 -> [w795 w799]
      tunnel: [w795 w798] -> _
      frame False {
      }
      frame True {
        n638 = Not(x=w797) -> (.not. x?=w796:bool)
        n639 = local write "Rectangle Tool"(w796) -> ()
        n640 = call "IMAGE ANALYSIS.vi"("Enum"=POST_ANALYSIS_ENUM."DRAW REC", "error in"=w799) -> ("error out"=w798:errorcluster)  [unwired: 8 in, 1 out]
      }
    }
    n641 = local read "SCAR MEASURMENT"() -> (w507:enum32{"Auto Scar", "Manual Scar"})
    n642 = local read "Fit to Screen Tool"() -> (w516:bool)
    n643 = local read "Resize Tool"() -> (w515:bool)
    n644 = case shown="\"Manual Scar\", Default" w507 {
      frame "Auto Scar" {
        n645 = property on="Cap Live Image" class="Bool (strict)"("BoolText.Text"="Report" ("Boolean Text.Text")) -> ()  [unwired: 2 in, 2 out]
      }
      frame "Manual Scar", Default {
        n646 = property on="Cap Live Image" class="Bool (strict)"("BoolText.Text"="Save Image" ("Boolean Text.Text")) -> ()  [unwired: 2 in, 2 out]
      }
    }
    n647 = local read "ROI Color Tool"() -> (w517:bool)
    n648 = local read "Pan Tool"() -> (w518:bool)
    n649 = case shown="True" w518 {
      selector: w518 -> [_ w785]
      tunnel: w514 -> [w783 w787]
      tunnel: [w783 w786] -> _
      frame False {
      }
      frame True {
        n650 = Not(x=w785) -> (.not. x?=w784:bool)
        n651 = call "IMAGE ANALYSIS.vi"("Enum"=POST_ANALYSIS_ENUM."PAN", "error in"=w787) -> ("error out"=w786:errorcluster)  [unwired: 8 in, 1 out]
        n652 = local write "Pan Tool"(w784) -> ()
      }
    }
    n653 = case shown="True" w515 {
      selector: w515 -> [_ w769]
      tunnel: w514 -> [w764 w766]
      tunnel: [w764 w765] -> _
      frame False {
      }
      frame True {
        n654 = Not(x=w769) -> (.not. x?=w768:bool)
        n655 = local write "Resize Tool"(w768) -> ()
        n656 = call "IMAGE ANALYSIS.vi"("Enum"=POST_ANALYSIS_ENUM."RESIZE MODE", "error in"=w766) -> ("error out"=w765:errorcluster)  [unwired: 8 in, 1 out]
      }
    }
    n657 = case shown="True" w516 {
      selector: w516 -> [_ w774]
      tunnel: [w770 w775] -> _
      tunnel: w514 -> [w770 w773]
      frame False {
      }
      frame True {
        n658 = Not(x=w774) -> (.not. x?=w772:bool)
        n659 = local write "Zoom Factore"(100.0 ("Zoom Factore")) -> ()
        n660 = local write "Fit to Screen Tool"(w772) -> ()
        n661 = call "IMAGE ANALYSIS.vi"("Enum"=POST_ANALYSIS_ENUM."FIT", "error in"=w773) -> ("error out"=w775:errorcluster)  [unwired: 8 in, 1 out]
      }
    }
    n662 = case shown="True" w517 {
      selector: w517 -> [_ w780]
      tunnel: [w777 w781] -> _
      tunnel: w514 -> [w777 w778]
      frame False {
      }
      frame True {
        n663 = Not(x=w780) -> (.not. x?=w779:bool)
        n664 = local write "ROI Color Tool"(w779) -> ()
        n665 = call "IMAGE ANALYSIS.vi"("Enum"=POST_ANALYSIS_ENUM."SET ROI COLOR", "error in"=w778) -> ("error out"=w781:errorcluster)  [unwired: 8 in, 1 out]
      }
    }
    n666 = local read "Quit"() -> (w531:bool)
  }
  n667 = property on="Service Password Log" class="Str"("Visible"=w12) -> ()  [unwired: 2 in, 2 out]
  n668 = property on="Password 3" class="Clust (strict)"("Visible"=w12) -> ()  [unwired: 2 in, 2 out]
  n669 = while {
    stop <- w865 stop-if-true
    n670 = local read "Image Path"() -> (w868:path)
    n671 = local read "Print 3"() -> (w871:bool)
    n672 = Equal?(x=w868, y=path "") -> (x = y?=w867:bool)
    n673 = Not(x=w867) -> (.not. x?=w866:bool)
    n674 = property on="Print 3" class="Bool (strict)"("Visible"=w866) -> ()  [unwired: 2 in, 2 out]
    n675 = case shown="True" w871 {
      frame False {
        n676 = local write "Rd"(TRUE ("Boolean 7")) -> ()
      }
      frame True {
        n677 = flat-sequence {
          tunnel: [w911] -> w879
          tunnel: [w898] -> w877
          tunnel: [w908] -> w873
          tunnel: w879 -> [w920]
          tunnel: [w920] -> w878
          tunnel: w877 -> [w919]
          tunnel: [w919] -> w876
          tunnel: [w917] -> w875
          tunnel: [w916] -> w874
          tunnel: w873 -> [w916]
          tunnel: w878 -> [w922]
          tunnel: w876 -> [w923]
          tunnel: w875 -> [_]
          tunnel: w874 -> [w921]
          frame #0 {
            n678 = case shown="True" "Rd" {
              frame False {
              }
              frame True {
                n679 = while {
                  tunnel: "abcdefABCDEF" ("string 2") -> [w890]
                  shift-right: [w888] -> w882
                  shift-left: "" -> [w887]
                  i -> [w897]
                  stop <- w896 stop-if-true
                  n680 = Random Number (0-1)() -> (number: 0 to 1=w891:dbl)
                  n681 = Multiply(x=w891, y=62.0) -> (x*y=w893:dbl)
                  n682 = Decrement(x="Length 2") -> (x-1=w886:i16)
                  n683 = To Word Integer(number=w893) -> (16bit integer=w894:i16)
                  n684 = String Subset(string=w890, offset (0)=w894, length (rest)=1 ("length (rest)")) -> (substring=w889:string)
                  n685 = Greater Or Equal?(x=w897, y=w886) -> (x >= y?=w896:bool)
                  n686 = Concatenate Strings(w889, w887) -> (w888:string)
                }
                "String 10" <- w882
                n687 = local write "Rd"(FALSE ("Boolean 7")) -> ()
              }
            }
          }
          frame #1 {
            w909 = "_resized.jpg" ("command line")
            (unwired) ".jpg -resize 320x240 " ("string")
            (unwired) "Choose an Image File" ("prompt")
            # "-resize 1798x425"
            n688 = local read "Image Path"() -> (w903:path)
            n689 = Strip Path(path=w903) -> (stripped path=w898:path, name=w899:string)
            n690 = Match Pattern(string=w899, regular expression=".jpg") -> (before substring=→"before substring 2":string, after substring=→"after substring":string)  [unwired: 1 in, 2 out]
            n691 = Match Pattern(string=w899, regular expression="\\") -> (before substring=w905:string)  [unwired: 1 in, 3 out]
            n692 = Match Pattern(string=w905, regular expression=".jpg") -> (before substring=w904:string)  [unwired: 1 in, 3 out]
            n693 = Concatenate Strings("cmd /c convert " ("string"), w904, ".jpg -resize 320x240  " ("command line"), w904, w909) -> (w912:string)
            n694 = call <vilib>:"System Exec.vi"("run minimized? (F)"=TRUE, "wait until completion? (T)"=TRUE, "working directory"=w898, "command line"=w912) -> ("error out"=w911:errorcluster)  [unwired: 4 in, 3 out]
            "error out 2" <- w911
            n695 = Concatenate Strings(w904, w909) -> (w908:string)
          }
          frame #2 {
            n696 = Wait (ms)(milliseconds to wait=u32 2000 ("millisecond timer value")) -> (millisecond timer value=w917:u32)
          }
          frame #3 {
            n697 = case shown="No Error" w922 {
              tunnel: w923 -> [w926 _]
              tunnel: w921 -> [w924 _]
              frame No Error {
                (unwired) ".jpg" ("string")
                n698 = Path To String(path=w926) -> (string=w930:string)
                n699 = Concatenate Strings(w930, "\\" ("string"), w924) -> (w929:string)
                n700 = String To Path(string=w929) -> (path=w928:path)
                n701 = call <vilib>:"Read JPEG File.vi"("path to JPEG file"=w928) -> ("image data"=w932:T11)  [unwired: 8 in, 2 out]
                "image data" <- w932
                n702 = local write "Print 3"(FALSE ("Print 2")) -> ()
                n703 = call <vilib>:"Draw Flattened Pixmap.vi"("image data"=w932) -> ("new picture"=→"new picture":picture)  [unwired: 8 in]
              }
              frame Error {
              }
            }
          }
        }
      }
    }
    n704 = Wait (ms)(milliseconds to wait=u32 20 ("millisecond timer value")) -> ()  [unwired: 1 out]
    n705 = local read "Quit"() -> (w865:bool)
  }
  n706 = while {
    tunnel: w33 -> [_]
    tunnel: w16 -> [_]
    stop <- w963 stop-if-true
    # "New Adv Logics"
    n707 = local read "Main Tab"() -> (w942:T2)
    n708 = local read "Main Tab"() -> (w961:T2)
    n709 = local read "Sign In"() -> (w960:bool)
    n710 = case shown="\"Adv Scar\"" w942 {
      frame "HOME", Default {
        n711 = local read "LIVE FEED MIN TEMP"() -> (w1090:bool)
        n712 = local write "LIVE FEED MAX TEMP"(TRUE ("LIVE FEED MAX TEMP")) -> ()
        n713 = local read "CAMERA ROI MIN TEMP"() -> (w1088:bool)
        n714 = case shown="True" w1090 {
          selector: w1090 -> [_ w1097]
          frame False {
          }
          frame True {
            n715 = Not(x=w1097) -> (.not. x?=w1096:bool)
            n716 = local write "LIVE FEED MIN TEMP"(w1096) -> ()
            n717 = call "CAMERA LIVE FEED FGV.vi"("Enum - Menu"=CAMERA_LIVE_FEED_ENUM."CAMERA MINIMIZE") -> ()  [unwired: 9 in, 2 out]
          }
        }
        n718 = case shown="True" w1088 {
          selector: w1088 -> [_ w1094]
          frame False {
          }
          frame True {
            n719 = Not(x=w1094) -> (.not. x?=w1093:bool)
            n720 = local write "CAMERA ROI MIN TEMP"(w1093) -> ()
            n721 = call "IMAGE ANALYSIS.vi"("Enum"=POST_ANALYSIS_ENUM."MINIMIZE UI") -> ()  [unwired: 9 in, 2 out]
          }
        }
        n722 = local write "CAMERA ROI MAX TEMP"(TRUE ("CAMERA ROI MAX TEMP")) -> ()
      }
      frame "Test Setup" {
        n723 = local read "LIVE FEED MIN TEMP"() -> (w1100:bool)
        n724 = local read "CAMERA ROI MIN TEMP"() -> (w1098:bool)
        n725 = local write "LIVE FEED MAX TEMP"(TRUE ("LIVE FEED MAX TEMP")) -> ()
        n726 = case shown="True" w1100 {
          selector: w1100 -> [_ w1107]
          frame False {
          }
          frame True {
            n727 = Not(x=w1107) -> (.not. x?=w1106:bool)
            n728 = local write "LIVE FEED MIN TEMP"(w1106) -> ()
            n729 = call "CAMERA LIVE FEED FGV.vi"("Enum - Menu"=CAMERA_LIVE_FEED_ENUM."CAMERA MINIMIZE") -> ()  [unwired: 9 in, 2 out]
          }
        }
        n730 = case shown="True" w1098 {
          selector: w1098 -> [_ w1104]
          frame False {
          }
          frame True {
            n731 = Not(x=w1104) -> (.not. x?=w1103:bool)
            n732 = local write "CAMERA ROI MIN TEMP"(w1103) -> ()
            n733 = call "IMAGE ANALYSIS.vi"("Enum"=POST_ANALYSIS_ENUM."MINIMIZE UI") -> ()  [unwired: 9 in, 2 out]
          }
        }
        n734 = local write "CAMERA ROI MAX TEMP"(TRUE ("CAMERA ROI MAX TEMP")) -> ()
      }
      frame "Acquire" {
        n735 = local read "LIVE FEED MIN TEMP"() -> (w1110:bool)
        n736 = local write "LIVE FEED MAX TEMP"(TRUE ("LIVE FEED MAX TEMP")) -> ()
        n737 = local read "CAMERA ROI MIN TEMP"() -> (w1108:bool)
        n738 = case shown="True" w1110 {
          selector: w1110 -> [_ w1117]
          frame False {
          }
          frame True {
            n739 = Not(x=w1117) -> (.not. x?=w1116:bool)
            n740 = local write "LIVE FEED MIN TEMP"(w1116) -> ()
            n741 = call "CAMERA LIVE FEED FGV.vi"("Enum - Menu"=CAMERA_LIVE_FEED_ENUM."CAMERA MINIMIZE") -> ()  [unwired: 9 in, 2 out]
          }
        }
        n742 = case shown="True" w1108 {
          selector: w1108 -> [_ w1114]
          frame False {
          }
          frame True {
            n743 = Not(x=w1114) -> (.not. x?=w1113:bool)
            n744 = local write "CAMERA ROI MIN TEMP"(w1113) -> ()
            n745 = call "IMAGE ANALYSIS.vi"("Enum"=POST_ANALYSIS_ENUM."MINIMIZE UI") -> ()  [unwired: 9 in, 2 out]
          }
        }
        n746 = local write "CAMERA ROI MAX TEMP"(TRUE ("CAMERA ROI MAX TEMP")) -> ()
      }
      frame "Adv Scar" {
        n747 = local read "CAMERA ROI MIN TEMP"() -> (w1118:bool)
        n748 = case shown="True" "LIVE FEED MAX TEMP" {
          selector: "LIVE FEED MAX TEMP" -> [_ w1139]
          frame False {
          }
          frame True {
            n749 = Not(x=w1139) -> (.not. x?=w1138:bool)
            n750 = local write "LIVE FEED MAX TEMP"(w1138) -> ()
            n751 = call "CAMERA LIVE FEED FGV.vi"("Enum - Menu"=CAMERA_LIVE_FEED_ENUM."CAMERA RESTORE") -> ("error out"=w1129:errorcluster)  [unwired: 9 in, 1 out]
            n752 = Type Cast(type=30, x=0) -> (*(type *) &x=w1133:i32)
            n753 = Add(x=w1133, y=48) -> (x+y=w1134:i32)
            n754 = call "CAMERA LIVE FEED FGV.vi"("Enum - Menu"=CAMERA_LIVE_FEED_ENUM."CAMERA MODE SET", "error in (no error)"=w1129, "CAMERA MODE"=w1134) -> ("error out"=w1126:errorcluster)  [unwired: 7 in, 1 out]
            n755 = call "CAMERA LIVE FEED FGV.vi"("Enum - Menu"=CAMERA_LIVE_FEED_ENUM."CAMERA GRAY", "error in (no error)"=w1126) -> ("error out"=w1125:errorcluster)  [unwired: 8 in, 1 out]
            n756 = call "LIST FILE NAMES.vi"("error in (no error)"=w1125) -> ("error out"=w1135:errorcluster, "filenames"=w1136:string[])  [unwired: 9 in]
            n757 = property on="FILE 3" class="CmbBox"(error in=w1135, "Strings[]"=w1136) -> ()  [unwired: 1 in, 2 out]
          }
        }
        n758 = case shown="True" w1118 {
          selector: w1118 -> [_ w1124]
          frame False {
          }
          frame True {
            n759 = Not(x=w1124) -> (.not. x?=w1123:bool)
            n760 = local write "CAMERA ROI MIN TEMP"(w1123) -> ()
            n761 = call "IMAGE ANALYSIS.vi"("Enum"=POST_ANALYSIS_ENUM."MINIMIZE UI") -> ()  [unwired: 9 in, 2 out]
          }
        }
        n762 = local write "CAMERA ROI MAX TEMP"(TRUE ("CAMERA ROI MAX TEMP")) -> ()
        "LIVE FEED MIN TEMP" <- TRUE ("LIVE FEED MIN TEMP")
      }
      frame "Adv Scar Report" {
        n763 = local read "CAMERA ROI MAX TEMP"() -> (w1140:bool)
        n764 = local read "LIVE FEED MIN TEMP"() -> (w1142:bool)
        n765 = local write "LIVE FEED MAX TEMP"(TRUE ("LIVE FEED MAX TEMP")) -> ()
        n766 = case shown="True" w1142 {
          selector: w1142 -> [_ w1151]
          frame False {
          }
          frame True {
            n767 = Not(x=w1151) -> (.not. x?=w1150:bool)
            n768 = local write "LIVE FEED MIN TEMP"(w1150) -> ()
            n769 = call "CAMERA LIVE FEED FGV.vi"("Enum - Menu"=CAMERA_LIVE_FEED_ENUM."CAMERA MINIMIZE") -> ()  [unwired: 9 in, 2 out]
          }
        }
        n770 = case shown="True" w1140 {
          selector: w1140 -> [_ w1148]
          frame False {
          }
          frame True {
            n771 = Not(x=w1148) -> (.not. x?=w1146:bool)
            n772 = local write "CAMERA ROI MAX TEMP"(w1146) -> ()
            n773 = call "IMAGE ANALYSIS.vi"("Enum"=POST_ANALYSIS_ENUM."SHOW UI") -> ("error out"=w1145:errorcluster)  [unwired: 9 in, 1 out]
            n774 = call "LIST FILE NAMES.vi"("error in (no error)"=w1145) -> ("filenames"=w1144:string[])  [unwired: 9 in, 1 out]
            n775 = property on="Test File List :" class="CmbBox"("Strings[]"=w1144) -> ()  [unwired: 2 in, 2 out]
          }
        }
        n776 = local write "CAMERA ROI MIN TEMP"(TRUE ("CAMERA ROI MIN TEMP")) -> ()
      }
      frame "Compare Files" {
        n777 = local read "LIVE FEED MIN TEMP"() -> (w1154:bool)
        n778 = local write "LIVE FEED MAX TEMP"(TRUE ("LIVE FEED MAX TEMP")) -> ()
        n779 = local read "CAMERA ROI MIN TEMP"() -> (w1152:bool)
        n780 = case shown="True" w1154 {
          selector: w1154 -> [_ w1161]
          frame False {
          }
          frame True {
            n781 = Not(x=w1161) -> (.not. x?=w1160:bool)
            n782 = local write "LIVE FEED MIN TEMP"(w1160) -> ()
            n783 = call "CAMERA LIVE FEED FGV.vi"("Enum - Menu"=CAMERA_LIVE_FEED_ENUM."CAMERA MINIMIZE") -> ()  [unwired: 9 in, 2 out]
          }
        }
        n784 = case shown="True" w1152 {
          selector: w1152 -> [_ w1158]
          frame False {
          }
          frame True {
            n785 = Not(x=w1158) -> (.not. x?=w1157:bool)
            n786 = local write "CAMERA ROI MIN TEMP"(w1157) -> ()
            n787 = call "IMAGE ANALYSIS.vi"("Enum"=POST_ANALYSIS_ENUM."MINIMIZE UI") -> ()  [unwired: 9 in, 2 out]
          }
        }
        n788 = local write "CAMERA ROI MAX TEMP"(TRUE ("CAMERA ROI MAX TEMP")) -> ()
      }
      frame "About" {
        n789 = local read "LIVE FEED MIN TEMP"() -> (w1164:bool)
        n790 = local write "LIVE FEED MAX TEMP"(TRUE ("LIVE FEED MAX TEMP")) -> ()
        n791 = local read "CAMERA ROI MIN TEMP"() -> (w1163:bool)
        n792 = case shown="True" w1164 {
          selector: w1164 -> [_ w1171]
          frame False {
          }
          frame True {
            n793 = Not(x=w1171) -> (.not. x?=w1170:bool)
            n794 = local write "LIVE FEED MIN TEMP"(w1170) -> ()
            n795 = call "CAMERA LIVE FEED FGV.vi"("Enum - Menu"=CAMERA_LIVE_FEED_ENUM."CAMERA MINIMIZE") -> ()  [unwired: 9 in, 2 out]
          }
        }
        n796 = case shown="True" w1163 {
          selector: w1163 -> [_ w1168]
          frame False {
          }
          frame True {
            n797 = Not(x=w1168) -> (.not. x?=w1167:bool)
            n798 = local write "CAMERA ROI MIN TEMP"(w1167) -> ()
            n799 = call "IMAGE ANALYSIS.vi"("Enum"=POST_ANALYSIS_ENUM."MINIMIZE UI") -> ()  [unwired: 9 in, 2 out]
          }
        }
        n800 = local write "CAMERA ROI MAX TEMP"(TRUE ("CAMERA ROI MIN TEMP")) -> ()
      }
      frame "Advance" {
        n801 = local read "LIVE FEED MIN TEMP"() -> (w1174:bool)
        n802 = local write "LIVE FEED MAX TEMP"(TRUE ("LIVE FEED MAX TEMP")) -> ()
        n803 = local read "CAMERA ROI MIN TEMP"() -> (w1172:bool)
        n804 = case shown="True" w1174 {
          selector: w1174 -> [_ w1181]
          frame False {
          }
          frame True {
            n805 = Not(x=w1181) -> (.not. x?=w1180:bool)
            n806 = local write "LIVE FEED MIN TEMP"(w1180) -> ()
